vi "Empty.vi"(8 "error in (no error)":errorcluster, 11 "Parameter to Hardware Map in":refnum<class "Parameter to Hardware Map.lvclass">) -> (0 "error out":errorcluster, 2 "Empty?":bool, 3 "Parameter to Hardware Map out":refnum<class "Parameter to Hardware Map.lvclass">)   [LabVIEW 2020, in "RxnRover.lvlib" / "Parameter to Hardware Map.lvclass"]
doc: "Test if the container is empty."
uses:
  Parameter to Hardware Map.lvclass
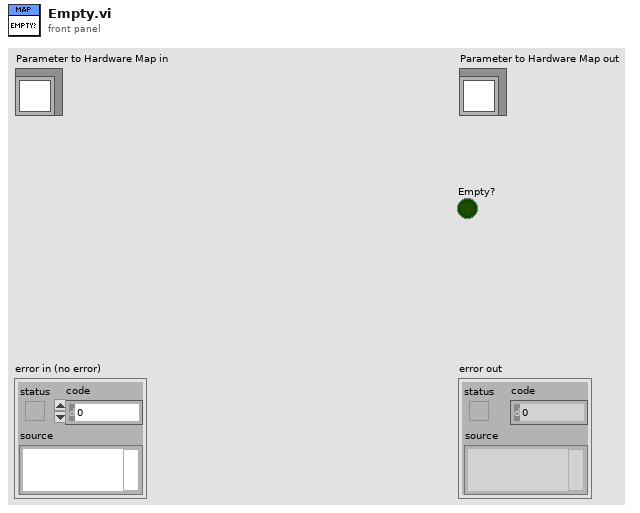
[diagram p1: front panel]
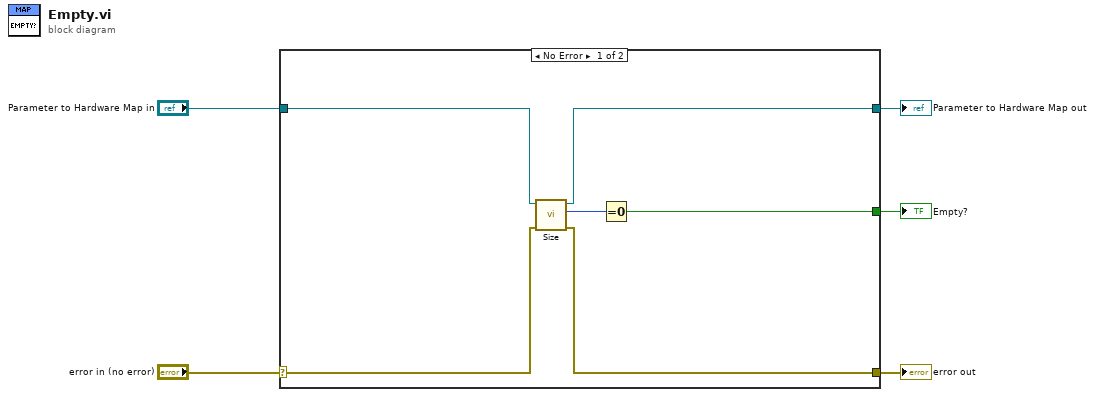
[diagram p0: block diagram]
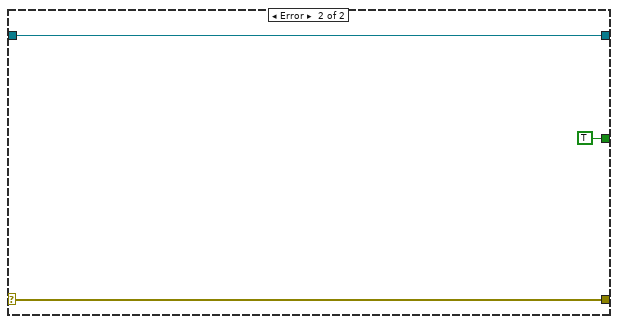
[diagram p2: hidden frame]
diagram:
  n1 = case shown="No Error" "error in (no error)" {
    selector: "error in (no error)" -> [w11 w14]
    tunnel: [w10 w14] -> w4
    tunnel: [w8 w13] -> w2
    tunnel: "Parameter to Hardware Map in" -> [w9 w13]
    tunnel: [w6 TRUE] -> w1
    frame No Error {
      n2 = call "Size.vi"("error in (no error)"=w11, "Parameter to Hardware Map in"=w9) -> ("error out"=w10:errorcluster, "Size"=w7:i32, "Parameter to Hardware Map out"=w8:refnum<class "Parameter to Hardware Map.lvclass">)  [unwired: 7 in]
      n3 = Equal To 0?(x=w7) -> (x = 0?=w6:bool)
    }
    frame Error {
    }
  }
  "error out" <- w4
  "Parameter to Hardware Map out" <- w2
  "Empty?" <- w1
